vi "RSZVB Set Vector Mixer Mode.vi"(8 "error in (no error)":errorcluster {"code" format="%.0x"}, 9 "Mixer Mode (0)":i32(ring) items=["Vector Mixer Measurement", "Frequency Conversion Off"], 10 "Channel (1)":i32=1, 11 "VISA session":refnum<visa-resource-name>) -> (0 "error out":errorcluster {"code" format="%.0x"}, 3 "dup VISA session":refnum<visa-resource-name>)   [LabVIEW 2011]
doc: "This VI toggle between the (frequency-converting) vector mixer mode and normal operation, where the analyzer measures the unconverted fundamental wave.\n\nRemote-control command(s):\n[SENSe<Ch>:]FREQuency:CONVersion VMIXer | FUNDamental"
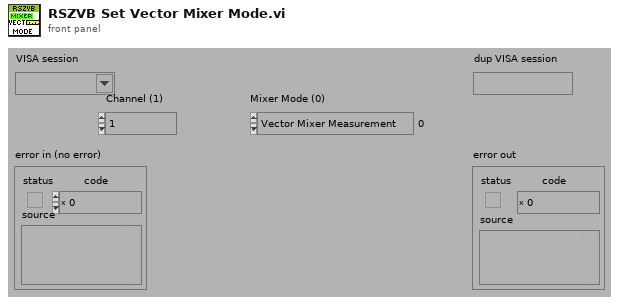
[diagram p1: front panel]
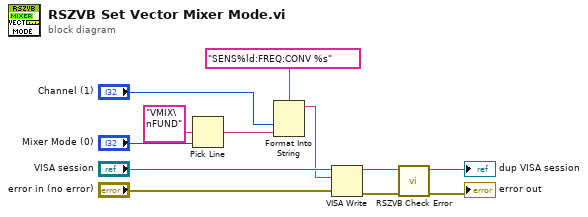
[diagram p0: block diagram]
diagram:
  n1 = Pick Line(multi-line string="VMIX\nFUND", line index="Mixer Mode (0)") -> (output string=w9:string)  [unwired: 1 in]
  n2 = Format Into String(format string="SENS%ld:FREQ:CONV %s", "Channel (1)", w9) -> (resulting string=w5:string)  [unwired: 2 in, 1 out]
  n3 = VISA Write(VISA resource name="VISA session", write buffer=w5, error in (no error)="error in (no error)") -> (VISA resource name out=w3:refnum<visa-resource-name>, error out=w4:errorcluster)  [unwired: 1 out]
  n4 = call "RSZVB Check Error.vi"("error in (no error)"=w4, "VISA session"=w3) -> ("error out"=→"error out":errorcluster, "dup VISA session"=→"dup VISA session":refnum<visa-resource-name>)  [unwired: 8 in]
